vi "Save_interim_img_png.vi"() -> ()   [LabVIEW 2020]
uses:
  <vilib>/vision/NI_Vision_Development_Module.lvlib
panel:
  out "Elapsed time [ms]":u32
  in  "h":i32=10 min=1 max=5000 step=1
  in  "w":i32=1 min=1 max=5000 step=1
  out "error out":errorcluster
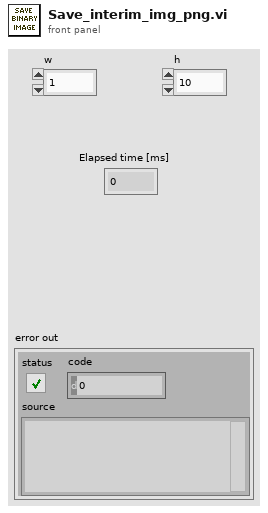
[diagram p1: front panel]
types:
  T1 = typedef "Image Type" = u32
  T2 = typedef "IMAQ Image.ctl" = refnum<image>
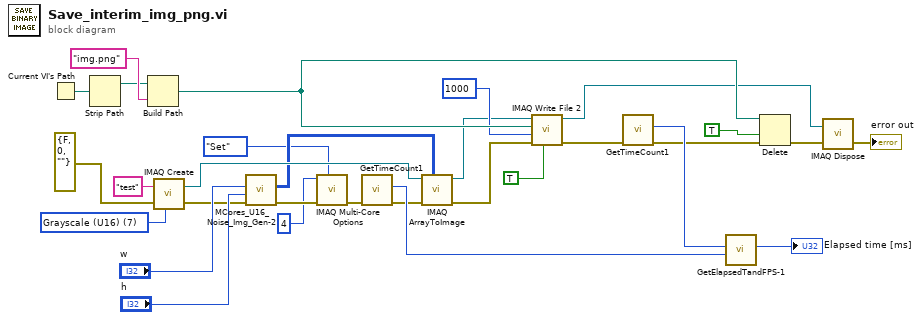
[diagram p0: block diagram]
diagram:
  w18 = T1 7 items=["Grayscale (U8)", "Grayscale (I16)", "Grayscale (SGL)", "Complex (CSG)", "RGB (U32)", "HSL (U32)", "RGB (U64)", "Grayscale (U16)"] ("Image Type")
  n1 = Current VI's Path() -> (path=w30:path)
  n2 = Strip Path(path=w30) -> (stripped path=w28:path)  [unwired: 1 out]
  n3 = Build Path(base path=w28, name or relative path="img.png" ("string")) -> (appended path=w14:path)
  n4 = call "IMAQ Create"("Image Name"="test", "Image Type"=w18, "error in (no error)"=errorcluster {"status"=FALSE, "code"=0, "source"=""}) -> ("New Image"=w9:T2, "error out"=w19:errorcluster)  [unwired: 2 in]
  n5 = call "MCores_U16_Noise_Img_Gen-2.vi"("error IN"=w19, "[IN] Width"="h", "[IN] Height"="w") -> ("error OUT"=w4:errorcluster, "[OUT] U16 Pixel Img"=w8:u16[][])  [unwired: 7 in]
  n6 = call "IMAQ Multi-Core Options"("Get/Set Number of Cores (Get)"=enum32{"Get", "Set", "Set Max Available"}."Set", "error in (no error)"=w4, "Specified Number of Cores"=u32 4) -> ("error out"=w3:errorcluster)  [unwired: 7 in, 1 out]
  n7 = call "GetTimeCount1.vi"("error IN"=w3) -> ("error OUT"=w11:errorcluster, "[OUT] Timer Count"=w24:u32)  [unwired: 9 in]
  n8 = call "IMAQ ArrayToImage"("Image Pixels (U16)"=w8, "error in (no error)"=w11, "Image"=w9) -> ("error out"=w10:errorcluster, "Image Out"=w7:T2)  [unwired: 7 in]
  n9 = call-poly "IMAQ Write File 2"("Use bit depth? (false)"=TRUE, "error in (no error)"=w10, "Image Quality"=u32 1000, "File Path"=w14, "Image"=w7) -> ("error out"=w6:errorcluster, "Image Out (duplicate)"=w5:T2)  [unwired: 5 in]
  n10 = call "GetTimeCount1.vi"("error IN"=w6) -> ("error OUT"=w22:errorcluster, "[OUT] Timer Count"=w25:u32)  [unwired: 9 in]
  n11 = call "GetElapsedTandFPS-1.vi"("[IN] Timer Count Before ALL [ms]"=w24, "[IN] Timer Count After ALL [ms]"=w25) -> ("[OUT] Elapsed time [ms]"=→"Elapsed time [ms]":u32)  [unwired: 3 in, 2 out]
  n12 = Delete(path (use dialog)=w14, confirm (F)=TRUE, error in=w22) -> (error out=w16:errorcluster)  [unwired: 2 in, 2 out]
  n13 = call "IMAQ Dispose"("Image"=w5, "error in (no error)"=w16) -> ("error out"=→"error out":errorcluster)  [unwired: 4 in]
